vi "3.1.8-Midbrain Act functional Global.vi"(1 "4.1- Midbrain Act Data":T1, 2 "Command":T2(ring)) -> (0 "4.1- Outputted Midbrain Act Data":T1)   [LabVIEW 2010]
uses:
  4-High Neurons/4.1-Midbrain Act Data.ctl
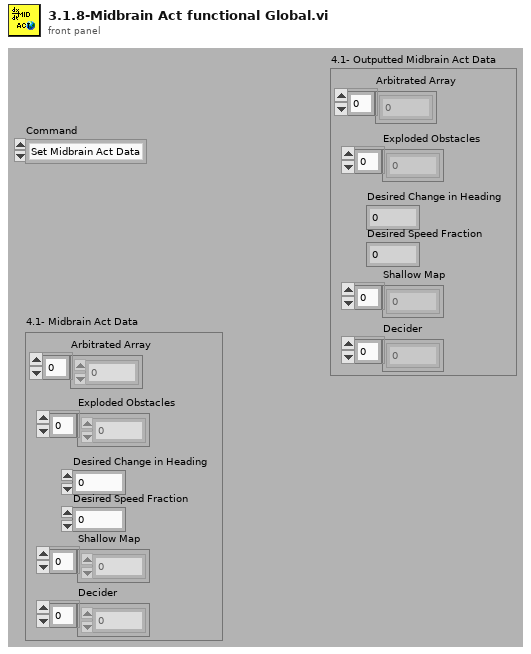
[diagram p1: front panel]
types:
  T1 = typedef "4.1-Midbrain Act Data.ctl" = cluster{"Arbitrated Array":sgl[], "Exploded Obstacles":sgl[], "Desired Change in Heading":sgl, "Desired Speed Fraction":sgl, "Shallow Map":dbl[], "Decider":dbl[]}
  T2 = enum16{"Set Midbrain Act Data", "Read Midbrain Act Data"}
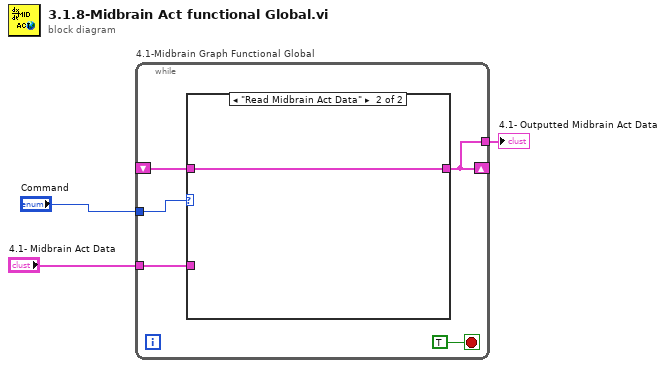
[diagram p0: block diagram]
diagram:
  n1 = while "4.1-Midbrain Graph Functional Global" {
    shift-right: [w4] -> _
    shift-left: _ -> [w5]
    tunnel: "Command" -> [w7]
    tunnel: "4.1- Midbrain Act Data" -> [w6]
    tunnel: [w4] -> w1
    stop <- TRUE stop-if-true
    n2 = case shown="\"Read Midbrain Act Data\"" w7 {
      tunnel: [w9 w10] -> w4
      tunnel: w6 -> [w9 _]
      tunnel: w5 -> [_ w10]
      frame "Set Midbrain Act Data", Default {
      }
      frame "Read Midbrain Act Data" {
      }
    }
  }
  "4.1- Outputted Midbrain Act Data" <- w1
